vi "类型3一组自动测试.vi"(11 "测试值":i32) -> ()   [LabVIEW 2010]
uses:
  全局量/试验配置信息.vi
  全局量/自动测试结果.vi
panel:
  out "D_IN_3":string[][](table) caption="表格"
  out "结束？":bool
  in  "同步_2":i32
  in  "同步_1":i32
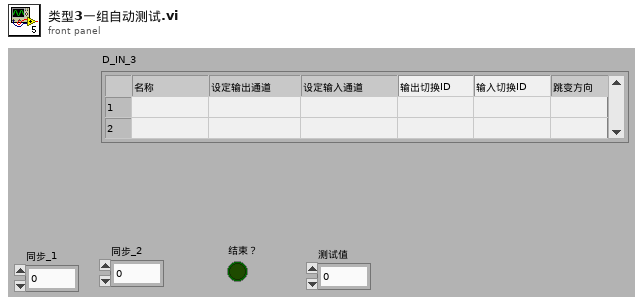
[diagram p1: front panel]
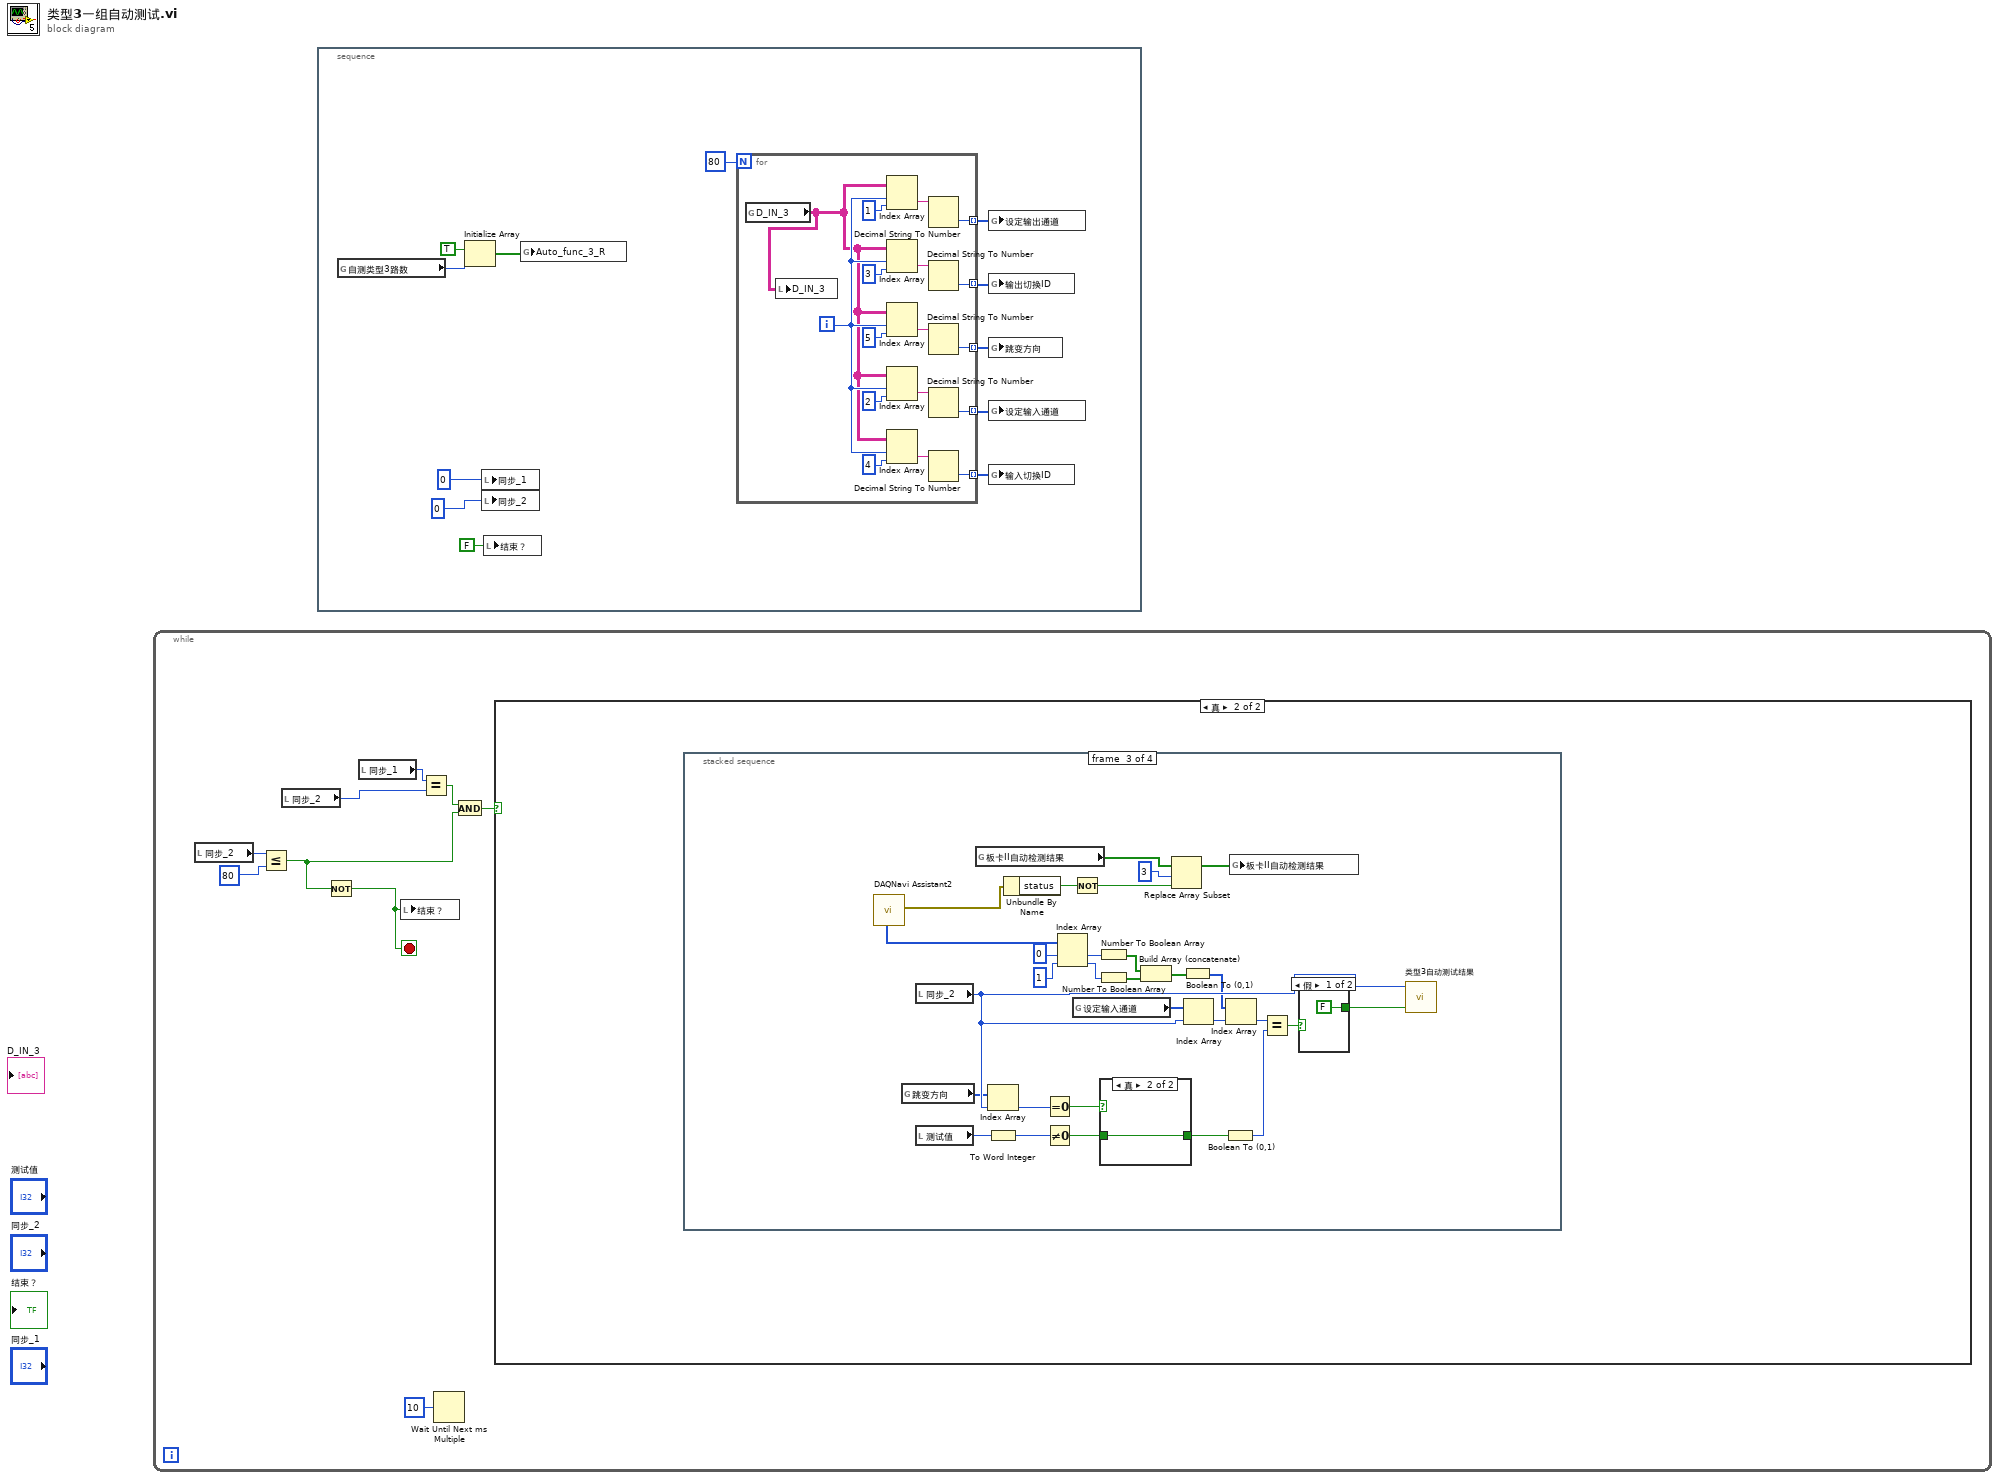
[diagram p0: block diagram]
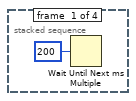
[diagram p3: hidden frame]
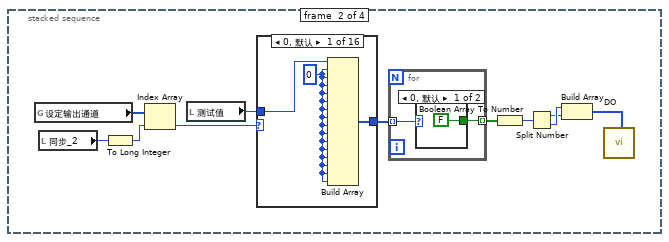
[diagram p4: hidden frame]
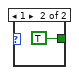
[diagram p5: hidden frame]
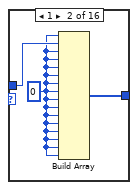
[diagram p6: hidden frame]
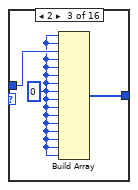
[diagram p7: hidden frame]
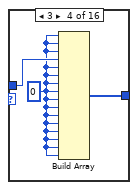
[diagram p8: hidden frame]
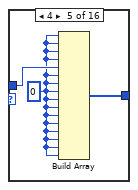
[diagram p9: hidden frame]
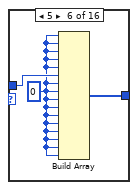
[diagram p10: hidden frame]
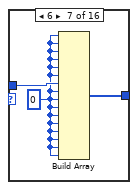
[diagram p11: hidden frame]
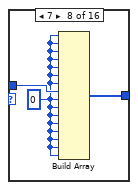
[diagram p12: hidden frame]
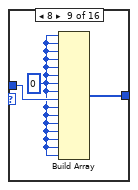
[diagram p13: hidden frame]
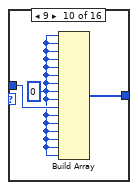
[diagram p14: hidden frame]
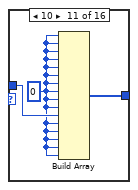
[diagram p15: hidden frame]
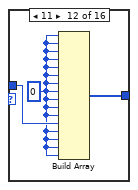
[diagram p16: hidden frame]
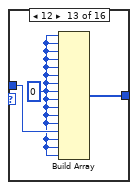
[diagram p17: hidden frame]
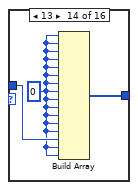
[diagram p18: hidden frame]
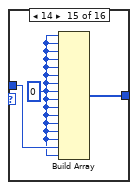
[diagram p19: hidden frame]
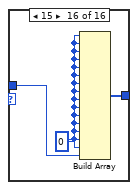
[diagram p20: hidden frame]
diagram:
  n1 = while {
    stop <- w1 stop-if-true
    n2 = local read "同步_2"() -> (w4:i32)
    n3 = Less Or Equal?(x=w4, y=80) -> (x <= y?=w5:bool)
    n4 = local read "同步_2"() -> (w2:i32)
    n5 = Not(x=w5) -> (.not. x?=w1:bool)
    n6 = local read "同步_1"() -> (w8:i32)
    n7 = local write "结束？"(w1) -> ()
    n8 = Equal?(x=w8, y=w2) -> (x = y?=w6:bool)
    n9 = Wait Until Next ms Multiple(millisecond multiple=u32 10 ("毫秒倍数")) -> ()  [unwired: 1 out]
    n10 = And(x=w6, y=w5) -> (x .and. y?=w7:bool)
    n11 = case shown="真" w7 {
      frame False {
      }
      frame True {
        n12 = stacked-sequence {
          frame #0 {
            n13 = Wait Until Next ms Multiple(millisecond multiple=u32 200 ("毫秒倍数")) -> ()  [unwired: 1 out]
          }
          frame #1 {
            n14 = global read "试验配置信息.vi" "设定输出通道"() -> (w21:i32[])
            n15 = local read "同步_2"() -> (w11:i32)
            n16 = To Long Integer(number=w11) -> (32bit integer=w13:i32)
            n17 = Index Array(array=w21, index=w13) -> (element=w20:i32)
            n18 = local read "测试值"() -> (w12:i32)
            n19 = case shown="0, 默认" w20 {
              tunnel: w12 -> [w28 w31 w33 w36 w39 w42 w45 w48 w51 w54 w57 w60 w63 w66 w69 w72]
              tunnel: [w27 w30 w34 w37 w40 w43 w46 w49 w52 w55 w58 w61 w64 w67 w70 w73] -> w14
              frame 0, Default {
                w26 = 0 ("y")
                n20 = Build Array(w28, w26, w26, w26, w26, w26, w26, w26, w26, w26, w26, w26, w26, w26, w26, w26) -> (w27:i32[])
              }
              frame 1 {
                w29 = 0 ("y")
                n21 = Build Array(w29, w31, w29, w29, w29, w29, w29, w29, w29, w29, w29, w29, w29, w29, w29, w29) -> (w30:i32[])
              }
              frame 2 {
                w32 = 0 ("y")
                n22 = Build Array(w32, w32, w33, w32, w32, w32, w32, w32, w32, w32, w32, w32, w32, w32, w32, w32) -> (w34:i32[])
              }
              frame 3 {
                w35 = 0 ("y")
                n23 = Build Array(w35, w35, w35, w36, w35, w35, w35, w35, w35, w35, w35, w35, w35, w35, w35, w35) -> (w37:i32[])
              }
              frame 4 {
                w38 = 0 ("y")
                n24 = Build Array(w38, w38, w38, w38, w39, w38, w38, w38, w38, w38, w38, w38, w38, w38, w38, w38) -> (w40:i32[])
              }
              frame 5 {
                w41 = 0 ("y")
                n25 = Build Array(w41, w41, w41, w41, w41, w42, w41, w41, w41, w41, w41, w41, w41, w41, w41, w41) -> (w43:i32[])
              }
              frame 6 {
                w44 = 0 ("y")
                n26 = Build Array(w44, w44, w44, w44, w44, w44, w45, w44, w44, w44, w44, w44, w44, w44, w44, w44) -> (w46:i32[])
              }
              frame 7 {
                w47 = 0 ("y")
                n27 = Build Array(w47, w47, w47, w47, w47, w47, w47, w48, w47, w47, w47, w47, w47, w47, w47, w47) -> (w49:i32[])
              }
              frame 8 {
                w50 = 0 ("y")
                n28 = Build Array(w50, w50, w50, w50, w50, w50, w50, w50, w51, w50, w50, w50, w50, w50, w50, w50) -> (w52:i32[])
              }
              frame 9 {
                w53 = 0 ("y")
                n29 = Build Array(w53, w53, w53, w53, w53, w53, w53, w53, w53, w54, w53, w53, w53, w53, w53, w53) -> (w55:i32[])
              }
              frame 10 {
                w56 = 0 ("y")
                n30 = Build Array(w56, w56, w56, w56, w56, w56, w56, w56, w56, w56, w57, w56, w56, w56, w56, w56) -> (w58:i32[])
              }
              frame 11 {
                w59 = 0 ("y")
                n31 = Build Array(w59, w59, w59, w59, w59, w59, w59, w59, w59, w59, w59, w60, w59, w59, w59, w59) -> (w61:i32[])
              }
              frame 12 {
                w62 = 0 ("y")
                n32 = Build Array(w62, w62, w62, w62, w62, w62, w62, w62, w62, w62, w62, w62, w63, w62, w62, w62) -> (w64:i32[])
              }
              frame 13 {
                w65 = 0 ("y")
                n33 = Build Array(w65, w65, w65, w65, w65, w65, w65, w65, w65, w65, w65, w65, w65, w66, w65, w65) -> (w67:i32[])
              }
              frame 14 {
                w68 = 0 ("y")
                n34 = Build Array(w68, w68, w68, w68, w68, w68, w68, w68, w68, w68, w68, w68, w68, w68, w69, w68) -> (w70:i32[])
              }
              frame 15 {
                w71 = 0 ("y")
                n35 = Build Array(w71, w71, w71, w71, w71, w71, w71, w71, w71, w71, w71, w71, w71, w71, w71, w72) -> (w73:i32[])
              }
            }
            n36 = for {
              tunnel: w14 -> [w23] mode=indexing
              tunnel: [w22] -> w19 mode=indexing
              n37 = case shown="0, 默认" w23 {
                tunnel: [FALSE TRUE] -> w22
                frame 0, Default {
                }
                frame 1 {
                }
              }
            }
            n38 = Boolean Array To Number ("布尔数组至数值转换")(Boolean array=w19) -> (number=w18:u16)
            n39 = Split Number(x=w18) -> (hi(x)=w15:u8, lo(x)=w16:u8)
            n40 = Build Array(w16, w15) -> (w17:u8[])
            n41 = call "DO"("dataIn(U8Array)"=w17) -> ()  [unwired: 2 in, 17 out]
          }
          frame #2 {
            n42 = call "DAQNavi Assistant2"() -> ("error out"=w76:errorcluster, "dataOut(U8Array)"=w100:u8[])  [unwired: 2 in, 16 out]
            n43 = global read "试验配置信息.vi" "跳变方向"() -> (w95:i32[])
            n44 = local read "同步_2"() -> (w101:i32)
            n45 = local read "测试值"() -> (w102:i32)
            n46 = global read "试验配置信息.vi" "板卡II自动检测结果"() -> (w77:bool[])
            n47 = Index Array(array=w95, index=w101) -> (element=w94:i32)
            n48 = To Word Integer ("转换为双字节整型")(number=w102) -> (16bit integer=w96:i16)
            n49 = Unbundle By Name(w76) -> ("status"=w75:bool)
            n50 = Equal To 0?(x=w94) -> (x = 0?=w93:bool)
            n51 = Not Equal To 0?(x=w96) -> (x != 0?=w92:bool)
            n52 = Index Array(array=w100, index #1=0 ("索引"), index #2=1 ("索引")) -> (element #1=w85:u8, element #2=w86:u8)
            n53 = Not(x=w75) -> (.not. x?=w74:bool)
            n54 = global read "试验配置信息.vi" "设定输入通道"() -> (w80:i32[])
            n55 = Number To Boolean Array(number=w85) -> (Boolean array=w81:bool[])
            n56 = Number To Boolean Array(number=w86) -> (Boolean array=w82:bool[])
            n57 = case shown="真" w93 {
              tunnel: w92 -> [w106 w107]
              tunnel: [w105 w107] -> w91
              frame False {
                n58 = Not(x=w106) -> (.not. x?=w105:bool)
              }
              frame True {
              }
            }
            n59 = Build Array (concatenate)(w81, w82) -> (w87:bool[])
            n60 = Replace Array Subset(array=w77, new element=w74, index=3 ("索引")) -> (w78:bool[])
            n61 = Boolean To (0,1) ("布尔值至(0,1)转换")(Boolean=w87) -> (0, 1=w88:i16[])
            n62 = Index Array(array=w80, index=w101) -> (element=w89:i32)
            n63 = Boolean To (0,1)(Boolean=w91) -> (0, 1=w90:i16)
            n64 = Index Array(array=w88, index=w89) -> (element=w97:i16)
            n65 = global write "试验配置信息.vi" "板卡II自动检测结果"(w78) -> ()
            n66 = Equal?(x=w97, y=w90) -> (x = y?=w98:bool)
            n67 = case shown="假" w98 {
              tunnel: [FALSE TRUE] -> w99
              frame False {
              }
              frame True {
              }
            }
            n68 = call "类型3自动测试结果.vi"("合格?"=w99, "第几组"=w101) -> ()  [unwired: 10 in]
          }
          frame #3 {
            n69 = local read "同步_1"() -> (w109:i32)
            n70 = local read "同步_2"() -> (w111:i32)
            n71 = Increment(x=w109) -> (x+1=w108:i32)
            n72 = Increment(x=w111) -> (x+1=w110:i32)
            n73 = local write "同步_2"(w110) -> ()
            n74 = local write "同步_1"(w108) -> ()
          }
        }
      }
    }
  }
  n75 = stacked-sequence {
    frame #0 {
      n76 = global read "试验配置信息.vi" "自测类型3路数"() -> (w113:i32)
      n77 = Initialize Array(TRUE ("元素"), w113) -> (w112:bool[])
      n78 = local write "同步_1"(0 ("同步_1")) -> ()
      n79 = local write "同步_2"(0 ("同步_1")) -> ()
      n80 = local write "结束？"(FALSE ("结束？")) -> ()
      n81 = global write "自动测试结果.vi" "Auto_func_3_R"(w112) -> ()
      n82 = for {
        N: 80 -> [_]
        tunnel: [w138] -> w116 mode=indexing
        tunnel: [w135] -> w117 mode=indexing
        tunnel: [w132] -> w118 mode=indexing
        tunnel: [w129] -> w119 mode=indexing
        tunnel: [w125] -> w120 mode=indexing
        i -> [w127]
        n83 = global read "试验配置信息.vi" "D_IN_3"() -> (w124:string[][])
        n84 = local write "D_IN_3"(w124) -> ()
        n85 = Index Array(array=w124, index (row)=w127, index (col)=1 ("禁用的索引 (列)")) -> (element=w137:string)
        n86 = Index Array(array=w124, index (row)=w127, index (col)=3 ("禁用的索引 (列)")) -> (element=w133:string)
        n87 = Index Array(array=w124, index (row)=w127, index (col)=5 ("禁用的索引 (列)")) -> (element=w126:string)
        n88 = Index Array(array=w124, index (row)=w127, index (col)=2 ("禁用的索引 (列)")) -> (element=w139:string)
        n89 = Index Array(array=w124, index (row)=w127, index (col)=4 ("禁用的索引 (列)")) -> (element=w130:string)
        n90 = Decimal String To Number(string=w137) -> (number=w135:i32)  [unwired: 2 in, 1 out]
        n91 = Decimal String To Number(string=w133) -> (number=w132:i32)  [unwired: 2 in, 1 out]
        n92 = Decimal String To Number(string=w126) -> (number=w125:i32)  [unwired: 2 in, 1 out]
        n93 = Decimal String To Number(string=w139) -> (number=w138:i32)  [unwired: 2 in, 1 out]
        n94 = Decimal String To Number(string=w130) -> (number=w129:i32)  [unwired: 2 in, 1 out]
      }
      n95 = global write "试验配置信息.vi" "设定输出通道"(w117) -> ()
      n96 = global write "试验配置信息.vi" "输出切换ID"(w118) -> ()
      n97 = global write "试验配置信息.vi" "跳变方向"(w120) -> ()
      n98 = global write "试验配置信息.vi" "设定输入通道"(w116) -> ()
      n99 = global write "试验配置信息.vi" "输入切换ID"(w119) -> ()
    }
  }
